vi "ParserTest.vi"   [LabVIEW 2010]
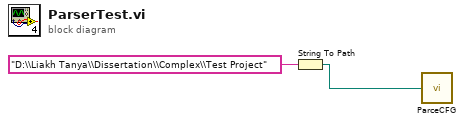
[diagram p0: block diagram]
diagram:
  n1 = String To Path(string="D:\\Liakh Tanya\\Dissertation\\Complex\\Test Project") -> (path=w1:path)
  n2 = call "ParceCFG.vi"("path"=w1) -> ()  [unwired: 1 in]
